vi "write_attributes.vi"(8 "error in (no error)":errorcluster, 10 "attributes":T1, 11 "RANSACRegressor in":refnum<class "RANSACRegressor.lvclass">) -> (0 "error out":errorcluster, 3 "RANSACRegressor out":refnum<class "RANSACRegressor.lvclass">)   [LabVIEW 2020, in "RANSACRegressor.lvclass"]
uses:
  RANSACRegressor.lvclass
  Controls/ransac_regressor_attributes.ctl
  RANSACRegressor.lvclass/RANSACRegressor.ctl
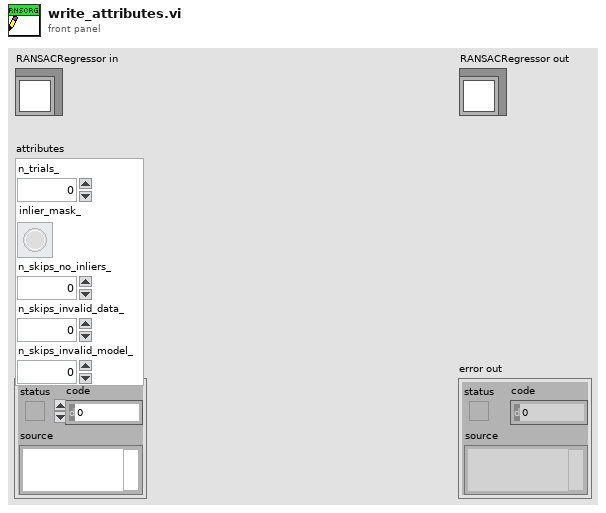
[diagram p1: front panel]
types:
  T1 = typedef "ransac_regressor_attributes.ctl" = cluster{"n_trials_":dbl, "inlier_mask_":bool[], "n_skips_no_inliers_":dbl, "n_skips_invalid_data_":dbl, "n_skips_invalid_model_":dbl}
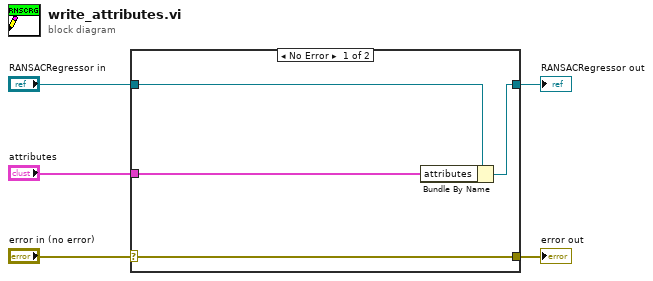
[diagram p0: block diagram]
diagram:
  n1 = case shown="No Error" "error in (no error)" {
    selector: "error in (no error)" -> [w9 w10]
    tunnel: [w9 w10] -> w4
    tunnel: [w7 w11] -> w2
    tunnel: "RANSACRegressor in" -> [w8 w11]
    tunnel: "attributes" -> [w6 _]
    frame No Error {
      n2 = Bundle By Name(cluster=w8, "attributes"=w6) -> (w7:refnum<class "RANSACRegressor.lvclass">)
    }
    frame Error {
    }
  }
  "error out" <- w4
  "RANSACRegressor out" <- w2
